vi "_emi_SMLoop Control Single.vi"(5 "Loop ID in":u16, 7 "Enable":bool, 9 "error in (no error)":errorcluster) -> (6 "Loop ID out":u16, 10 "error out":errorcluster)   [LabVIEW 2011]
doc: "Set the wanted execution state of a SMLoop."
uses:
  Loop control/Private/_emi_Loop control int action.ctl
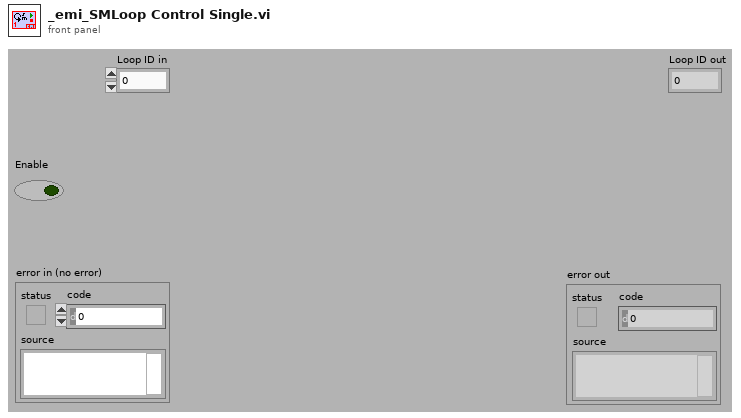
[diagram p1: front panel]
types:
  T1 = typedef "_emi_Loop control int action.ctl" = enum16{"Init index", "Get index", "Set index", "Get Size"}
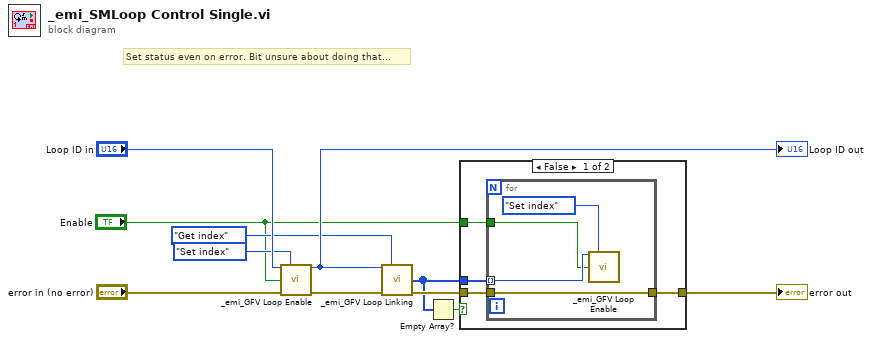
[diagram p0: block diagram]
diagram:
  # "Set status even on error. Bit unsure about doing that..."
  n1 = call "_emi_GFV Loop Enable.vi"("Loop Index/Numb"="Loop ID in", "Action(Get Index)"=_emi_Loop_control_int_action."Set index", "Loop enable In(T)"="Enable", "error in (no error)"="error in (no error)") -> ("Index out"=w6:u16, "error out"=w8:errorcluster)  [unwired: 8 in, 2 out]
  "Loop ID out" <- w6
  n2 = call "_emi_GFV Loop Linking.vi"("Loop Index/Numb"=w6, "Action(Get Index)"=_emi_Loop_control_int_action."Get index", "error in (no error)"=w8) -> ("Linked indexes out"=w2:u16[], "error out"=w3:errorcluster)  [unwired: 9 in, 2 out]
  n3 = Empty Array?(array=w2) -> (empty?=w4:bool)
  n4 = case shown="False" w4 {
    tunnel: w3 -> [w15 w20]
    tunnel: [w14 w20] -> w7
    tunnel: w2 -> [w13 _]
    tunnel: "Enable" -> [w12 _]
    frame False {
      n5 = for {
        tunnel: w15 -> [w19]
        tunnel: [w19] -> w14
        tunnel: w13 -> [w17] mode=indexing
        tunnel: w12 -> [w16]
        n6 = call "_emi_GFV Loop Enable.vi"("Loop Index/Numb"=w17, "Action(Get Index)"=_emi_Loop_control_int_action."Set index", "Loop enable In(T)"=w16) -> ()  [unwired: 9 in, 4 out]
      }
    }
    frame True {
      # "Empty"
    }
  }
  "error out" <- w7
